vi "YRPHfH.vi"(8 "error in (no error)":errorcluster, 11 "navX - Base in":refnum<class "navX - Base.lvclass">) -> (0 "error out":errorcluster, 3 "navX - Base out":refnum<class "navX - Base.lvclass">)   [LabVIEW 2015, in "navX Library v3.lvlib" / "navX - Base.lvclass"]
uses:
  navX - Base.lvclass
  navX - Base.lvclass/navX - Base.ctl
  navX Registry Cache/navX Registry Cache.lvclass
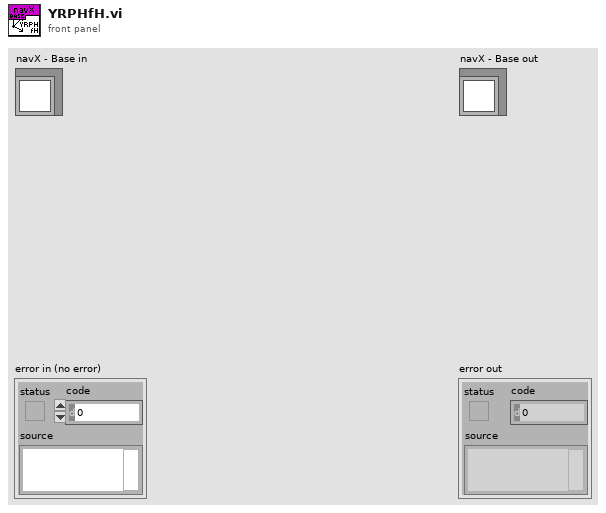
[diagram p1: front panel]
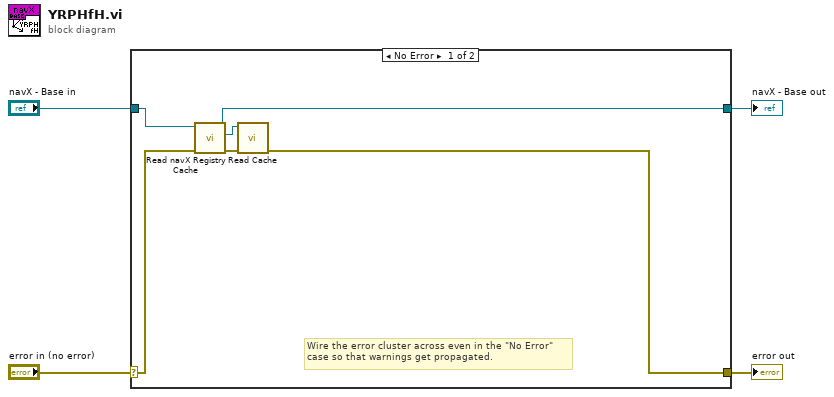
[diagram p0: block diagram]
diagram:
  n1 = case shown="No Error" "error in (no error)" {
    selector: "error in (no error)" -> [w9 w12]
    tunnel: [w5 w12] -> w3
    tunnel: [w6 w11] -> w1
    tunnel: "navX - Base in" -> [w10 w11]
    frame No Error {
      # "Wire the error cluster across even in the \"No Error\"\ncase so that warnings get propagated."
      n2 = call "Read navX Registry Cache.vi"("error in (no error)"=w9, "navX - Base in"=w10) -> ("error out"=w7:errorcluster, "navX Library v3.lvlib:navX Registry Cache.lvclass"=w8:refnum<class "navX Registry Cache.lvclass">, "navX - Base out"=w6:refnum<class "navX - Base.lvclass">)  [unwired: 7 in]
      n3 = call "Read Cache.vi"("error in (no error)"=w7, "navX Registry Cache in"=w8) -> ("error out"=w5:errorcluster)  [unwired: 7 in, 2 out]
    }
    frame Error {
    }
  }
  "error out" <- w3
  "navX - Base out" <- w1
